vi "Get Waveform Reference Channel.vi"(8 "error in (no error)":errorcluster, 11 "Reference in":waveform(dbl)) -> (0 "error out":errorcluster, 2 "Reference Channel":i32, 3 "Reference out":waveform(dbl))   [LabVIEW 2019, in "Instrument.Lockin.lvlib" / "Instrument.DAQ.lvclass"]
uses:
  Instrument.DAQ.lvclass
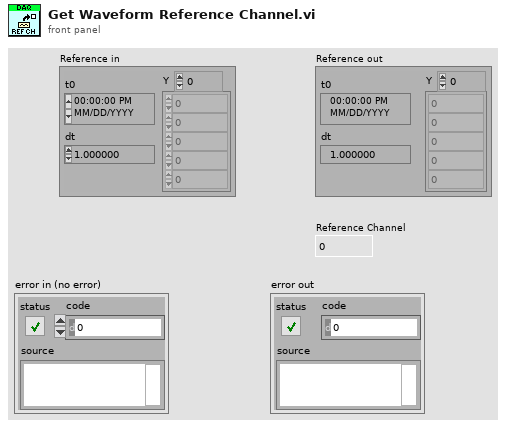
[diagram p1: front panel]
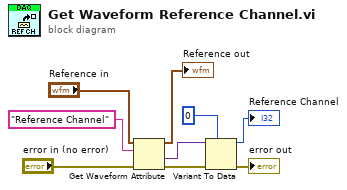
[diagram p0: block diagram]
diagram:
  n1 = Get Waveform Attribute(4:"error in (no error)", 6:"Reference Channel" ("name"), 7:"Reference in") -> (0:w2:errorcluster, 1:w3:variant, 3:→"Reference out":waveform(dbl))  [unwired: 1 in, 1 out]
  n2 = Variant To Data(error in=w2, type=0 ("Reference"), Variant=w3) -> (data=→"Reference Channel":i32, error out=→"error out":errorcluster)
